vi "SetHorizontal.vi"(4 "TriggerHoldoff":dbl, 5 "ViewportLength":dbl, 7 "SmartScope in":refnum<k24>) -> (0 "TrigSliderMin":dbl, 1 "TrigSliderMax":dbl, 3 "SmartScope out":refnum<k24>)   [LabVIEW 2019]
uses:
  C:/Program Files (x86)/LabNation/SmartScope/DeviceInterface.dll
  Program Files (x86)/LabNation/SmartScope/DeviceInterface.dll
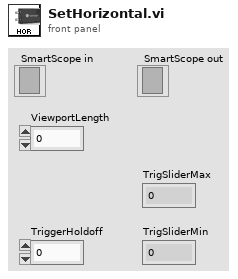
[diagram p1: front panel]
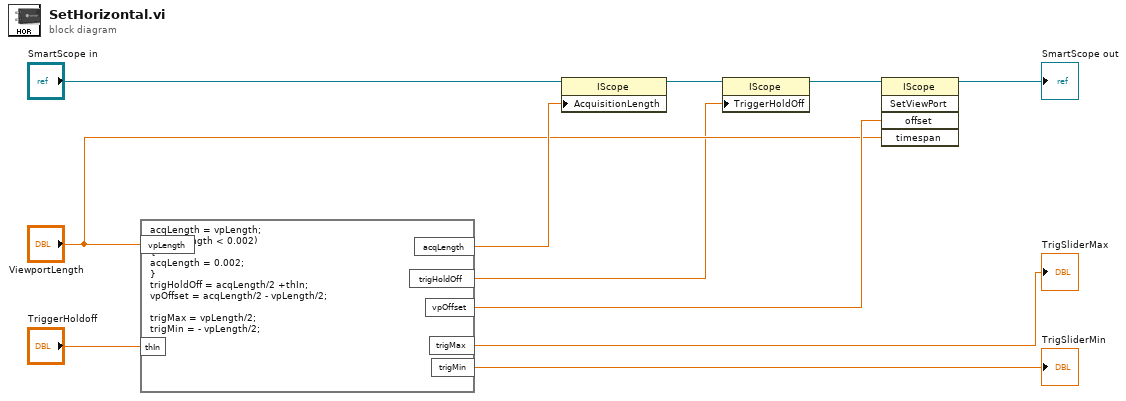
[diagram p0: block diagram]
diagram:
  n1 = formula code="acqLength = vpLength;\nif (acqLength < 0.002)\n{\nacqLength = 0.002;\n}\ntrigHoldOff = acqLength/2 +thIn;\nvpOffset = acqLength/2 - vpLength/2;\n\ntrigMax = vpLength/2;\ntrigMin = - vpLength/2;"("vpLength"="ViewportLength", "thIn"="TriggerHoldoff") -> ("acqLength"=w6:dbl, "trigHoldOff"=w3:dbl, "vpOffset"=w7:dbl, "trigMax"=→"TrigSliderMax":dbl, "trigMin"=→"TrigSliderMin":dbl)
  n2 = property class="IScope"(reference="SmartScope in", "AcquisitionLength"=w6) -> (reference out=w5:refnum<k24>)  [unwired: 1 in, 1 out]
  n3 = property class="IScope"(reference=w5, "TriggerHoldOff"=w3) -> (reference out=w8:refnum<k24>)  [unwired: 1 in, 1 out]
  n4 = invoke class="IScope" method="SetViewPort"(reference=w8, "offset"=w7, "timespan"="ViewportLength") -> (reference out=→"SmartScope out":refnum<k24>)  [unwired: 2 in, 4 out]
